vi "Snap control.vi"(0 "Variables in":T3, 1 "Snap in":bool, 2 "QBundle in":T2, 3 "Queue in":T1={"Enable zero"=FALSE, "Engr data [Unit]"=[], "Zero button"=FALSE, "Zero [V]"=[], "Timestamp [s]"=0.0, "Write sample"=FALSE, "Record control"=FALSE, "Stop"=FALSE, "error"={"status"=FALSE, "code"=0, "source"=""}, "Raw data [V]\n(all samples)"=[], "Raw data [V]"=[], "Loop count"=1, "Initial time [s]"=0.0, "Scale (0) & Offset (1)"=[], "Image count"=0.0} {"Initial time [s]" format="%_19f"; "Raw data [V]\n(all samples)" format="%0.2f"; "Timestamp [s]" format="%_19f"}) -> (4 "Snap out":bool, 5 "Variables out":T3, 6 "QBundle out":T2, 7 "Queue out":T1={"Enable zero"=FALSE, "Engr data [Unit]"=[], "Zero button"=FALSE, "Zero [V]"=[], "Timestamp [s]"=0.0, "Write sample"=FALSE, "Record control"=FALSE, "Stop"=FALSE, "error"={"status"=FALSE, "code"=0, "source"=""}, "Raw data [V]\n(all samples)"=[], "Raw data [V]"=[], "Loop count"=1, "Initial time [s]"=0.0, "Scale (0) & Offset (1)"=[], "Image count"=0.0} {"Initial time [s]" format="%_19f"; "Raw data [V]\n(all samples)" format="%0.2f"; "Timestamp [s]" format="%_19f"})   [LabVIEW 2020]
uses:
  Queue.ctl
  Constants.ctl
  QBundle.ctl
panel:
  # "Description: \nSnap control switches control on for single loop iteration.\nCases are outlined in associated documentation."
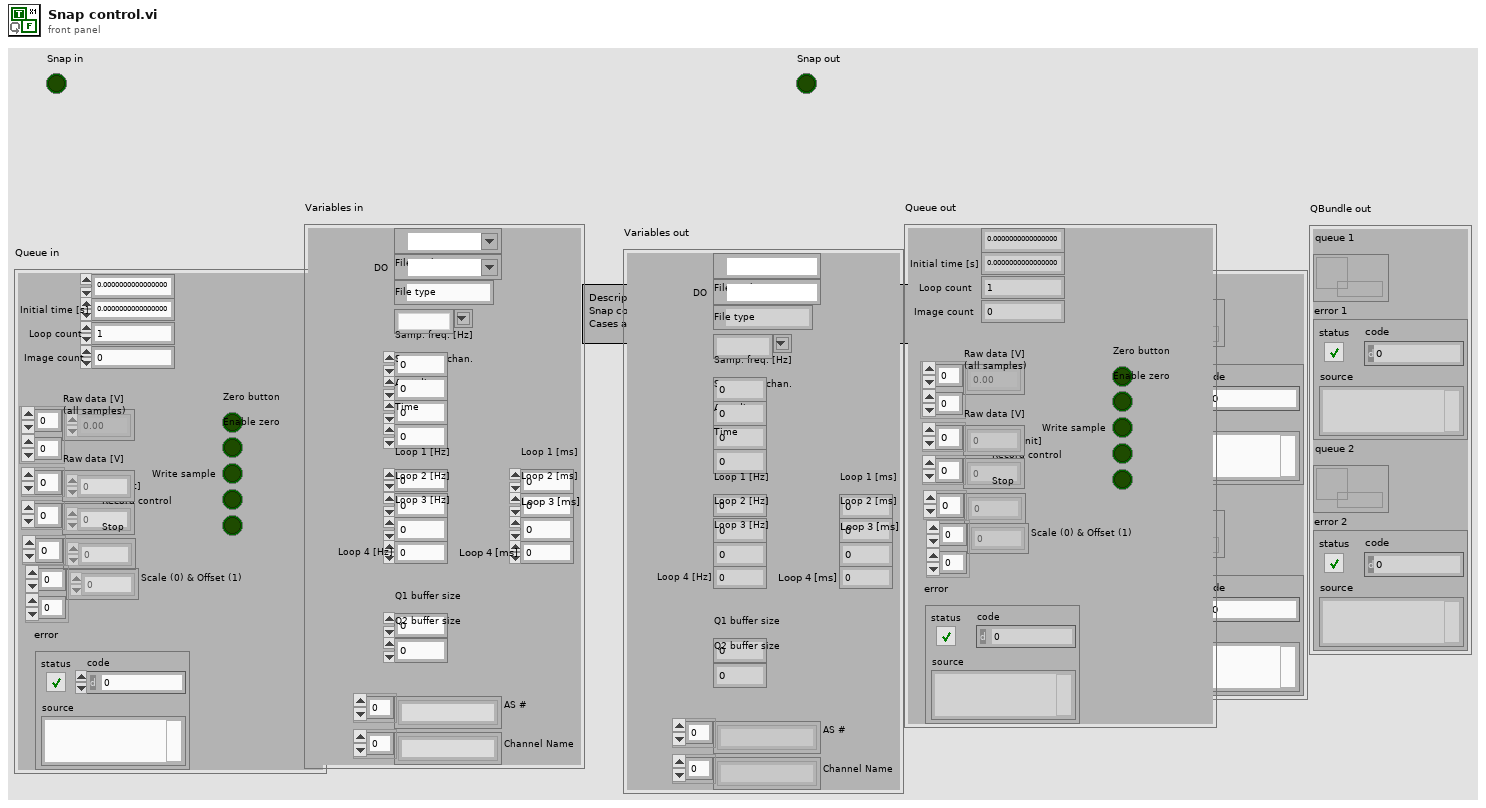
[diagram p1: front panel]
types:
  T1 = typedef "Queue.ctl" = cluster{"Enable zero":bool, "Engr data [Unit]":dbl[], "Zero button":bool, "Zero [V]":dbl[], "Timestamp [s]":dbl, "Write sample":bool, "Record control":bool, "Stop":bool, "error":errorcluster, "Raw data [V]\n(all samples)":dbl[][], "Raw data [V]":dbl[], "Loop count":i64, "Initial time [s]":dbl, "Scale (0) & Offset (1)":dbl[][], "Image count":dbl}
  T2 = typedef "QBundle.ctl" = cluster{"queue 1":refnum<queue>, "error 1":errorcluster, "queue 2":refnum<queue>, "error 2":errorcluster}
  T3 = typedef "Constants.ctl" = cluster{"Time":u16, "Samp. freq. [Hz]":dbl, "Samp. per chan.":i32, "Avg. div.":i32, "File path":path, "AI":refnum<k21>, "Loop 1 [Hz]":dbl, "Loop 2 [Hz]":dbl, "Loop 3 [Hz]":dbl, "Loop 1 [ms]":dbl, "Loop 2 [ms]":dbl, "Loop 3 [ms]":dbl, "Q1 buffer size":i32, "Q2 buffer size":i32, "File type":string, "Loop 4 [Hz]":dbl, "Loop 4 [ms]":dbl, "Channel Name":string[], "AS #":string[], "DO":refnum<k21>}
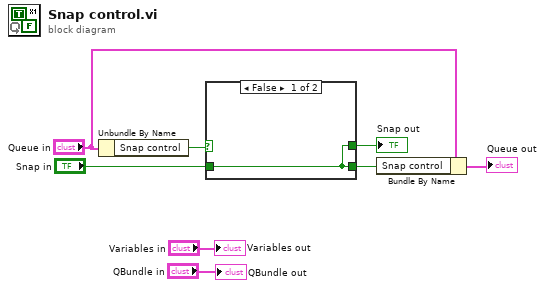
[diagram p0: block diagram]
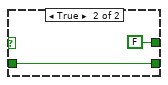
[diagram p2: hidden frame]
diagram:
  n1 = Unbundle By Name("Queue in") -> ("Snap control"=w3:bool)
  n2 = case shown="False" w3 {
    tunnel: [w9 FALSE] -> w6
    tunnel: [w9 w10] -> w5
    tunnel: "Snap in" -> [w9 w10]
    frame False {
    }
    frame True {
    }
  }
  "Snap out" <- w6
  n3 = Bundle By Name(cluster="Queue in", "Snap control"=w5) -> (→"Queue out":T1)
  "Variables out" <- "Variables in"
  "QBundle out" <- "QBundle in"
